vi "GUI.SelectPollTags.vi"(8 "error in":errorcluster, 10 "Refs":T1[](array[typedef]) format="%.0x", 11 "Parent Ref":T1=18446744073709551615 format="%.0x") -> (0 "error out":errorcluster, 1 "Cancelled?":bool, 2 "Refs out":T1[](array[typedef]) format="%.0x", 3 "Parent Ref Out":T1=18446744073709551615 format="%.0x")   [LabVIEW 2019, in "OPC UA Client System Explorer.lvlib"]
uses:
  OPC UA Client System Explorer.lvlib
  <vilib>/NI VeriStand/Custom Device API/Custom Device API.lvlib
  <vilib>/NI VeriStand/Custom Device Tools/Custom Device Utility Library/Custom Device Utility Library.lvlib
  <vilib>/NI VeriStand/Custom Device Tools/Custom Device Utility Library/NI VeriStand - Search for Item by GUID.vi
  <vilib>/NI VeriStand/Custom Device Tools/Custom Device Utility Library/Search Direction.ctl
  Shared/Constants.vi
  Shared/OPC UA Client Shared.lvlib
  <vilib>/NI VeriStand/Custom Device API/Custom Device Item Ref.ctl
  NationalInstruments.VeriStand.SystemStorageUI
panel:
  in  "Cancel":bool
  in  "OK":bool
  in  "TreeBrowserWF":refnum<k24>(container)
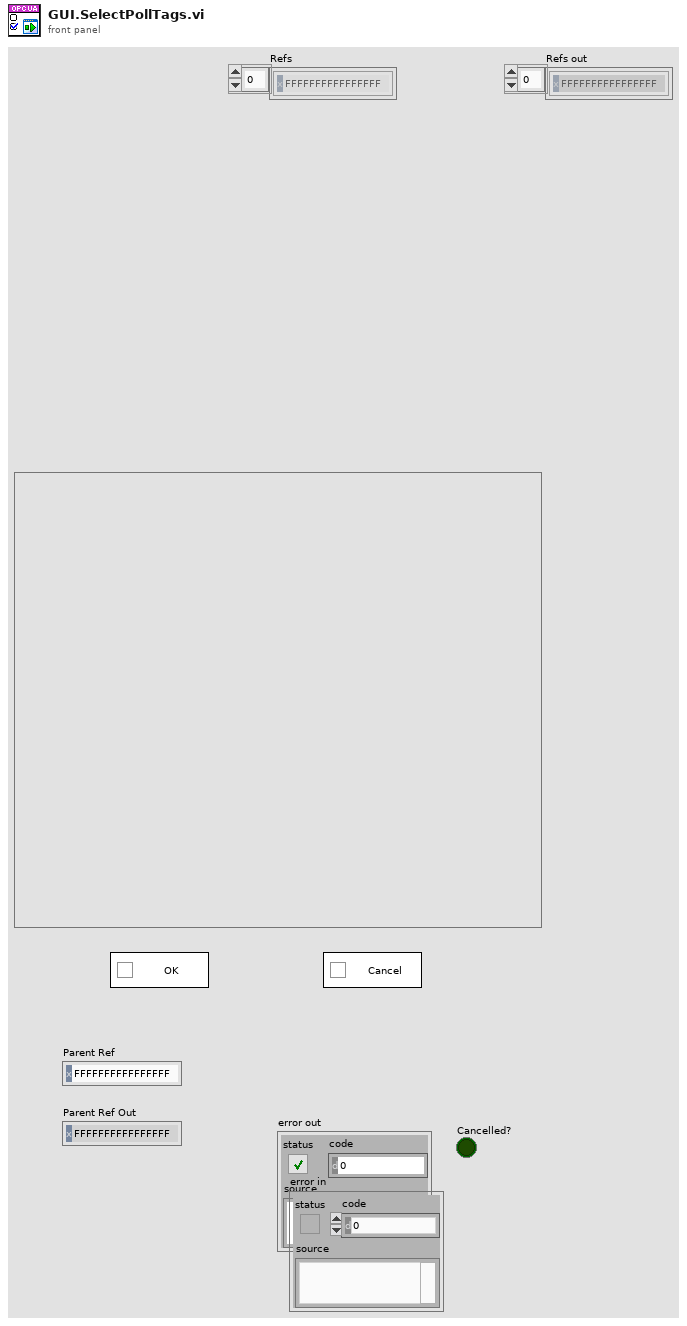
[diagram p1: front panel]
types:
  T1 = typedef "Custom Device API.lvlib/Custom Device Item Ref.ctl" = u64
  T2 = typedef "Custom Device Utility Library.lvlib/Search Direction.ctl" = enum16{"Down", "Up"}
  T3 = typedef "Custom Device API.lvlib/Custom Device Pointer.ctl" = refnum<k24>
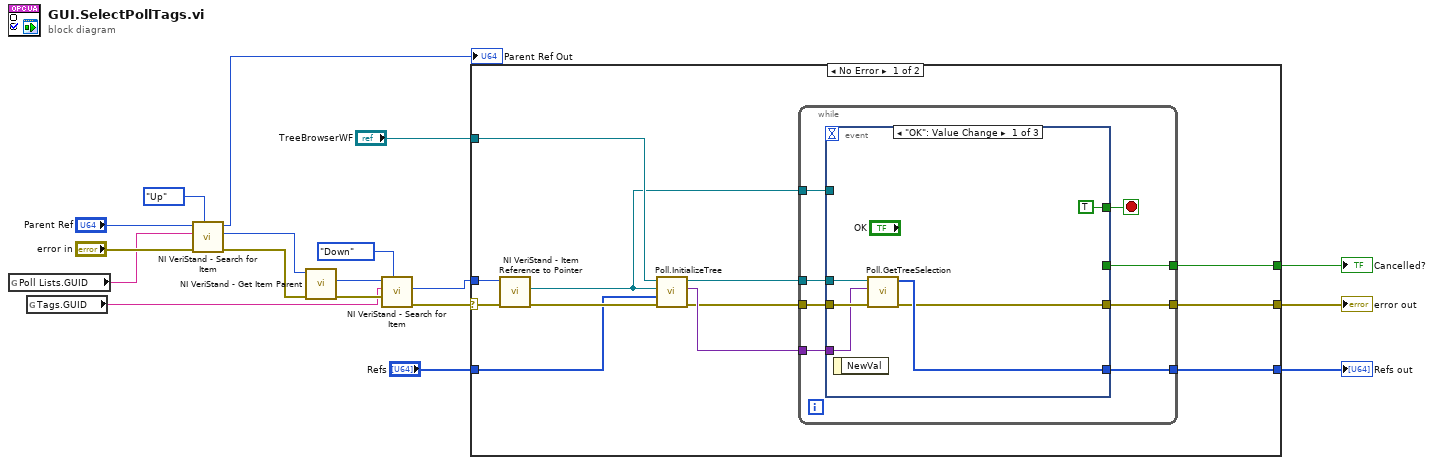
[diagram p0: block diagram]
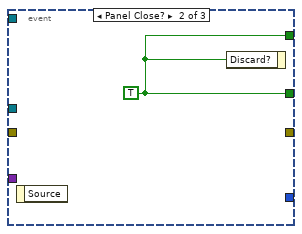
[diagram p2: hidden frame]
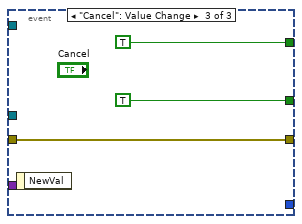
[diagram p3: hidden frame]
diagram:
  n1 = global read "Constants.vi" "Poll Lists.GUID"() -> (w10:string)
  n2 = global read "Constants.vi" "Tags.GUID"() -> (w3:string)
  n3 = call-poly <vilib>:"NI VeriStand - Search for Item.vi"("Direction (Down)"=Search_Direction."Up", "error in"="error in", "Item GUID"=w10, "Section Ref in"="Parent Ref") -> ("error out"=w6:errorcluster, "Item Ref"=w2:T1, "Section Ref out"=→"Parent Ref Out":T1)  [unwired: 4 in, 1 out]
  n4 = call <vilib>:"NI VeriStand - Get Item Parent.vi"("error in (no error)"=w6, "Item Ref in"=w2) -> ("error out"=w7:errorcluster, "Parent Ref"=w8:T1)  [unwired: 6 in, 2 out]
  n5 = call-poly <vilib>:"NI VeriStand - Search for Item.vi"("Direction (Down)"=Search_Direction."Down", "error in"=w7, "Item GUID"=w3, "Section Ref in"=w8) -> ("error out"=w5:errorcluster, "Item Ref"=w1:T1)  [unwired: 4 in, 2 out]
  n6 = case shown="No Error" w5 {
    selector: w5 -> [w29 w50]
    tunnel: "TreeBrowserWF" -> [w26 _]
    tunnel: w1 -> [w30 _]
    tunnel: [w28 _] -> w17
    tunnel: [w23 w50] -> w16
    tunnel: [w27 w49] -> w9
    tunnel: "Refs" -> [w20 w49]
    frame No Error {
      n7 = call <vilib>:"NI VeriStand - Item Reference to Pointer.vi"("error in (no error)"=w29, "Item Ref in"=w30) -> ("error out"=w22:errorcluster, "Node Pointer"=w19:T3)  [unwired: 6 in, 2 out]
      n8 = call "Poll.InitializeTree.vi"("error in (no error)"=w22, "Refs"=w20, "Node Pointer"=w19, "TreeBrowserRef"=w26) -> ("error out"=w21:errorcluster, "Channels"=w25:variant, "TreeBrowserRef 2"=w24:refnum<k24>)  [unwired: 5 in]
      n9 = while {
        tunnel: w21 -> [w38]
        tunnel: w24 -> [w37]
        tunnel: [w35] -> w28
        tunnel: [w34] -> w23
        tunnel: [w33] -> w27
        tunnel: w25 -> [w32]
        tunnel: w19 -> [w31]
        stop <- w36 stop-if-true
        n10 = event shown="[0] \"OK\": Value Change" {
          selector: _ -> [_ _ _]
          dyn-events: _ -> [_ _ _]
          timeout: _ -> [_ _ _]
          tunnel: w38 -> [w44 _ w48]
          tunnel: w37 -> [w43 _ _]
          tunnel: [w39 _ w48] -> w34
          tunnel: [TRUE w45 TRUE] -> w36
          tunnel: [_ w45 TRUE] -> w35
          tunnel: [w41 _ _] -> w33
          tunnel: w32 -> [w42 _ _]
          tunnel: w31 -> [_ _ _]
          event "OK": Value Change {
            n11 = event-data() -> ()  [unwired: 1 in, 1 out]
            n12 = call "Poll.GetTreeSelection.vi"("error in (no error)"=w44, "Input Channels"=w42, ".NET Refnum in"=w43) -> ("error out"=w39:errorcluster, "Refs"=w41:T1[])  [unwired: 7 in]
          }
          event Panel Close? {
            w45 = TRUE
            n13 = event-data() -> ()  [unwired: 1 in, 1 out]
            n14 = event-data("Discard?"=w45) -> ()  [unwired: 1 in, 1 out]
          }
          event "Cancel": Value Change {
            n15 = event-data() -> ()  [unwired: 1 in, 1 out]
          }
        }
      }
    }
    frame Error {
    }
  }
  "Cancelled?" <- w17
  "error out" <- w16
  "Refs out" <- w9
